vi "VI AK TCP - FTIR.vi"(6 "Aktionen":T1, 7 "connection ID":refnum<k5>, 8 "error in":errorcluster caption="error out", 9 "Port":u16=3615, 10 "IP-Adresse:":string, 11 "Fehlerzähler":i16) -> (0 "error out":errorcluster, 3 "Fehlerzähler":i16, 4 "Aktionen":T1, 5 "connection ID":refnum<k5>)   [LabVIEW 2020, in "FT-IR.lvlib" / "AK-Interface.lvlib"]
uses:
  AK-Interface.lvlib
  Aktionen AK.ctl
  Kommandos verwalten Aktionen.ctl
  TCP Timeout Aktionen - FTIR.ctl
  AK-Schnittstelle/AK-Schnittstelle.lvlib
  AK-Schnittstelle/Daten weitergeben Aktionen.ctl
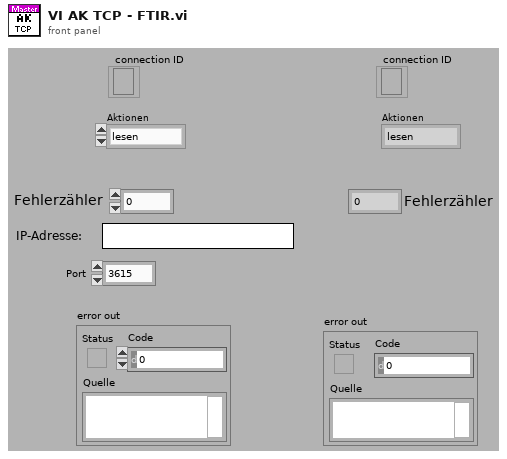
[diagram p1: front panel]
types:
  T1 = typedef "FT-IR.lvlib/AK-Interface.lvlib/Aktionen AK.ctl" = enum16{"lesen", "initialisieren", "beenden", "AK Komm"}
  T2 = typedef "FT-IR.lvlib/AK-Interface.lvlib/TCP Timeout Aktionen - FTIR.ctl" = enum16{"lesen", "setzen"}
  T3 = typedef "FT-IR.lvlib/AK-Interface.lvlib/Kommandos verwalten Aktionen.ctl" = enum16{"lesen", "setzen Ende", "setzen Pos1", "senden", "initalisieren", "prüfen", "Kommandos"}
  T4 = typedef "AK-Schnittstelle.lvlib/Daten weitergeben Aktionen.ctl" = enum16{"lesen", "schreiben", "Log löschen", "Detail", "Detail löschen", "AK FT-IR", "FT-IR löschen"}
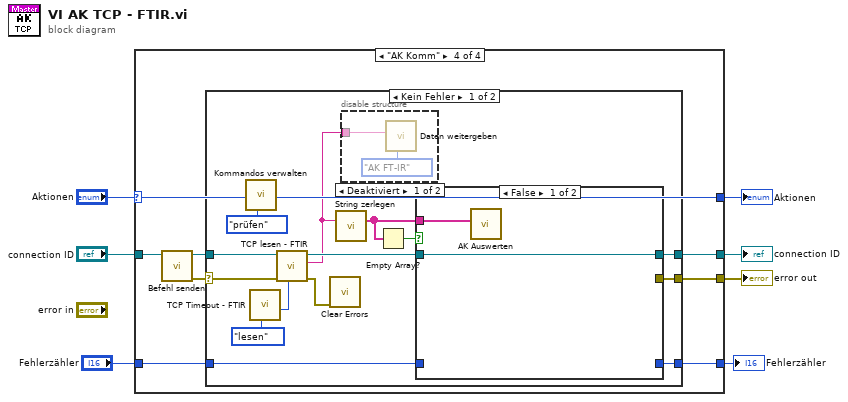
[diagram p0: block diagram]
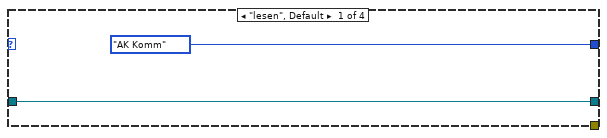
[diagram p2: hidden frame]
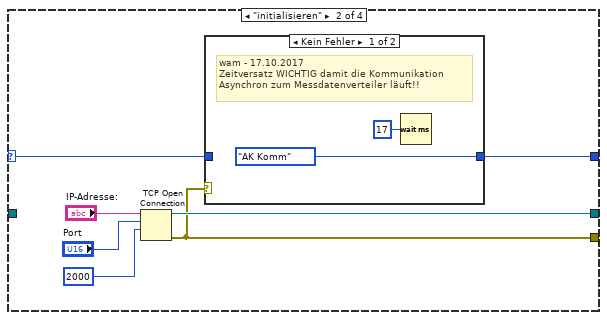
[diagram p3: hidden frame]
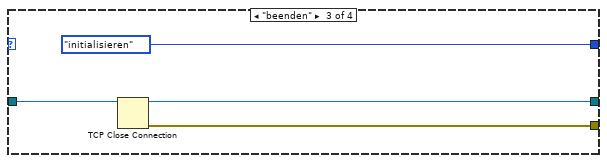
[diagram p5: hidden frame]
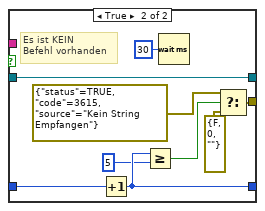
[diagram p7: hidden frame]
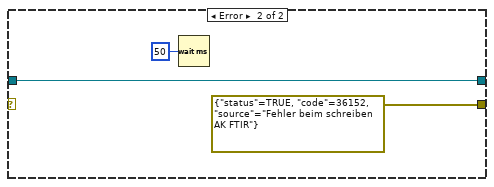
[diagram p8: hidden frame]
diagram:
  n1 = case shown="\"AK Komm\"" "Aktionen" {
    selector: "Aktionen" -> [_ w11 _ w26]
    tunnel: [_ w12 w23 w31] -> w6
    tunnel: [w9 w13 w21 w30] -> w4
    tunnel: "connection ID" -> [w9 _ w22 w29]
    tunnel: [Aktionen_AK."AK Komm" ("Aktionen") w10 Aktionen_AK."initialisieren" ("Aktionen") w26] -> w3
    tunnel: [_ _ _ w25] -> w1
    tunnel: "Fehlerzähler" -> [_ _ _ w24]
    frame "lesen", Default {
    }
    frame "initialisieren" {
      n2 = TCP Open Connection(address="IP-Adresse:", remote port or service name="Port", timeout ms (60000)=2000 ("timeout ms (wait forever: -1)")) -> (connection ID=w13:refnum<k5>, error out=w12:errorcluster)  [unwired: 2 in]
      n3 = case shown="Kein Fehler" w12 {
        tunnel: [Aktionen_AK."AK Komm" ("Aktionen") w19] -> w10
        tunnel: w11 -> [_ w19]
        frame No Error {
          # "wam - 17.10.2017\nZeitversatz WICHTIG damit die Kommunikation \nAsynchron zum Messdatenverteiler läuft!!"
          n4 = Wait (ms)(milliseconds to wait=u32 17 ("Zu wartende ms")) -> ()  [unwired: 1 out]
        }
        frame Error {
        }
      }
    }
    frame "beenden" {
      n5 = TCP Close Connection(connection ID=w22) -> (connection ID out=w21:refnum<k5>, error out=w23:errorcluster)  [unwired: 2 in]
    }
    frame "AK Komm" {
      n6 = call "Befehl senden.vi"("connection ID"=w29) -> ("error out"=w27:errorcluster, "connection ID"=w28:refnum<k5>)  [unwired: 8 in, 1 out]
      n7 = case shown="Kein Fehler" w27 {
        selector: w27 -> [w36 _]
        tunnel: [w39 errorcluster {"status"=TRUE, "code"=36152, "source"="Fehler beim schreiben AK FTIR"} ("error out")] -> w31
        tunnel: [w42 w61] -> w30
        tunnel: w28 -> [w41 w61]
        tunnel: [w33 _] -> w25
        tunnel: w24 -> [w32 _]
        frame No Error {
          n8 = call "Kommandos verwalten.vi"("Aktionen"=Kommandos_verwalten_Aktionen."prüfen") -> ()  [unwired: 8 in, 3 out]
          n9 = call "TCP Timeout - FTIR.vi"("Aktionen Timeout"=TCP_Timeout_Aktionen_-_FTIR."lesen") -> ("Timeout lesen"=w35:i32)  [unwired: 9 in, 1 out]
          n10 = call "TCP lesen - FTIR.vi"("Timeout"=w35, "Fehler (Eingang)"=w36, "connection ID"=w41) -> ("error out"=w34:errorcluster, "Daten (Ausgang)"=w37:string, "connection ID"=w43:refnum<k5>)  [unwired: 6 in]
          n11 = call <vilib>:"Clear Errors.vi"("error in (no error)"=w34) -> ()  [unwired: 5 in, 2 out]
          n12 = call "String zerlegen.vi"("read buffer"=w37) -> ("Array"=w45:string[])  [unwired: 14 in]
          n13 = disable-structure shown="Deaktiviert" {
            disable-tunnel: w37 -> [w47 _]
            frame Disabled {
              n14 = call "Daten weitergeben.vi"("Aktionen"=Daten_weitergeben_Aktionen."AK FT-IR", 10:w47) -> ()  [unwired: 5 in, 5 out]
            }
            frame Enabled {
            }
          }
          n15 = Empty Array?(array=w45) -> (empty?=w44:bool)
          n16 = case shown="False" w44 {
            tunnel: w45 -> [w48 _]
            tunnel: w43 -> [w49 w58]
            tunnel: [w49 w58] -> w42
            tunnel: [_ w53] -> w39
            tunnel: [_ w55] -> w33
            tunnel: w32 -> [_ w56]
            frame False {
              n17 = call "AK Auswerten.vi"("Array"=w48) -> ()  [unwired: 11 in]
            }
            frame True {
              # "Es ist KEIN \nBefehl vorhanden"
              n18 = Increment(x=w56) -> (x+1=w55:i16)
              n19 = Greater Or Equal?(x=w55, y=i16 5) -> (x >= y?=w51:bool)
              n20 = Wait (ms)(milliseconds to wait=u32 30 ("Zu wartende ms")) -> ()  [unwired: 1 out]
              n21 = Select(t=errorcluster {"status"=TRUE, "code"=3615, "source"="Kein String Empfangen"} ("error out"), s=w51, f=errorcluster {"status"=FALSE, "code"=0, "source"=""}) -> (s? t:f=w53:errorcluster)
            }
          }
        }
        frame Error {
          n22 = Wait (ms)(milliseconds to wait=u32 50 ("Zu wartende ms")) -> ()  [unwired: 1 out]
        }
      }
    }
  }
  "error out" <- w6
  "connection ID" <- w4
  "Aktionen" <- w3
  "Fehlerzähler" <- w1
